vi "Configure TS DAC Results.vi"(8 "error in":errorcluster, 11 "Test Stand in":refnum<class "Heat Flow Test Stand.lvclass">) -> (0 "error out":errorcluster, 3 "Test Stand out":refnum<class "Heat Flow Test Stand.lvclass">)   [LabVIEW 2019, in "Test Stands.lvlib" / "Heat Flow Test Stand.lvclass"]
uses:
  Heat Flow Test Stand.lvclass
  Generic Test Stand/Generic Test Stand.lvclass
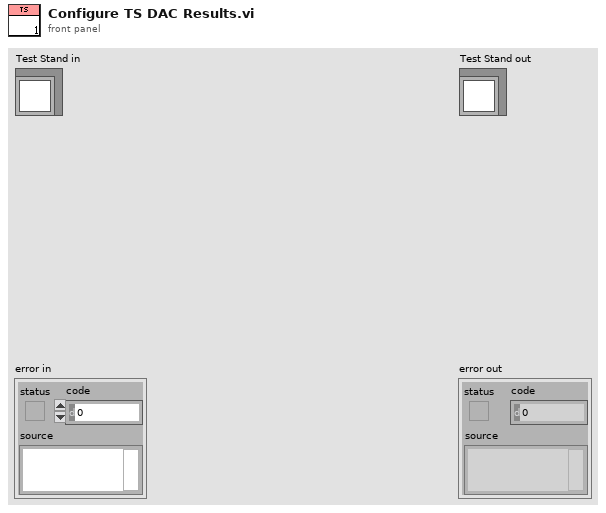
[diagram p1: front panel]
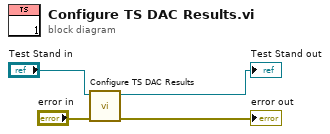
[diagram p0: block diagram]
diagram:
  n1 = call-parent "Configure TS DAC Results.vi"("error in"="error in", "Test Stand in"="Test Stand in") -> ("error out"=→"error out":errorcluster, "Test Stand out"=→"Test Stand out":refnum<class "Heat Flow Test Stand.lvclass">)  [unwired: 8 in]
